vi "dfd_Dummy_FIRCtrlUnit.vi"(1 "reset":bool, 2 "input valid":bool, 3 "coefSetIdx":u16) -> (5 "ready for input":bool, 7 "output valid":bool, 8 "opState":T1, 9 "coefRDAddr":u16)   [LabVIEW 2017]
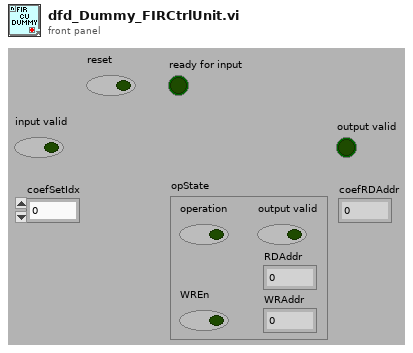
[diagram p1: front panel]
types:
  T1 = cluster{"operation":bool, "RDAddr":u16, "WREn":bool, "WRAddr":u16, "output valid":bool}
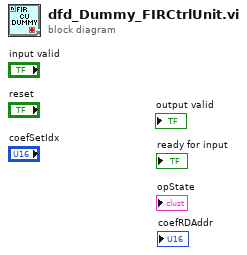
[diagram p0: block diagram]
diagram:
